vi "SPD.Liser Driver Test.vi"(8 "Error In":errorcluster, 11 "SPD.Stand Ctrl in":T1 {"spdDeviceSession"."hidSPD.Controller"."HV_bias" format="%#_6p, V"; "spdDeviceSession"."hidSPD.Controller"."TSet" format="%#_6p, DegC"}) -> (0 "Error Out":errorcluster, 1 "ok":bool, 2 "report":string, 3 "SPD.Stand Ctrl out":T1 {"spdDeviceSession"."hidSPD.Controller"."HV_bias" format="%#_6p, V"; "spdDeviceSession"."hidSPD.Controller"."TSet" format="%#_6p, DegC"})   [LabVIEW 2018]
uses:
  typedefs/SPD.Stand Ctrl.ctl
  Instruments/SPD HID Interface/hidSPDLibForLabView/LibVIs/hidSPD Controls/hidSPD Device Session.ctl
  Instruments/SPD HID Interface/hidSPDLibForLabView/LibVIs/hidSPD Controls/hidSPD Controller.ctl
  Instruments/KC705 DevBoard/typedefs/DevB.Session.ctl
  Instruments/KeySight 53230A/typedefs/FreqC.Session.ctl
  Instruments/KeySight 8164B/KeySight 8164B LAN InstrLib/typedefs/KeySight 8164B control.ctl
  Instruments/LeCroy SDA830/typedefs/LeCroy.Session.ctl
  typedefs/SPD.Events.ctl
  <vilib>/Utility/config.llb/Config Data RefNum.ctl
  typedefs/SPD.Meas Result.ctl
  Instruments/KeySight 8164B/KeySight 8164B LAN InstrLib/typedefs/KeySight 8164B Power Unit.ctl
  Instruments/KeySight 8164B/KeySight 8164B LAN InstrLib.lvlib
  Instruments/SPD HID Interface/hidSPDLibForLabView/hidSPDLibForLabView.lvlib
  <vilib>/Utility/config.llb/NI_LVConfig.lvlib
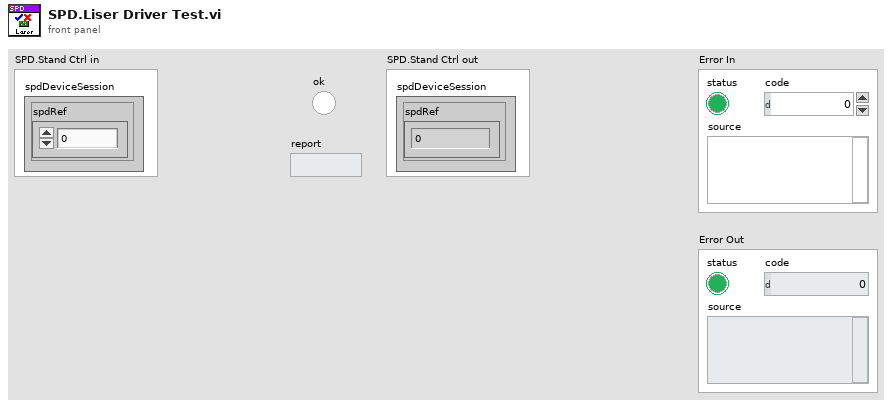
[diagram p1: front panel]
types:
  T1 = typedef "SPD.Stand Ctrl.ctl" = cluster{"spdDeviceSession":T2, "DevBSession":T4, "FreqCSession":T5, "8164BSession":T6, "LeCroySession":T7, "Events":T8, "configFile":T9, "SPD.Result":T10}
  T2 = typedef "hidSPDLibForLabView.lvlib/hidSPD Device Session.ctl" = cluster{"spdRef":u64, "connected":bool, "spdName":string, "hidSPD.Controller":T3}
  T3 = typedef "hidSPDLibForLabView.lvlib/hidSPD Controller.ctl" = cluster{"TSet":sgl, "HV_bias":sgl, "DDS_stb_code":u16}
  T4 = typedef "DevB.Session.ctl" = cluster{"DevBRef":refnum<visa-resource-name>, "connected":bool}
  T5 = typedef "FreqC.Session.ctl" = cluster{"FreqCRef":refnum<visa-resource-name>, "timeout":dbl, "Gate":dbl, "connected":bool}
  T6 = typedef "KeySight 8164B LAN InstrLib.lvlib/KeySight 8164B control.ctl" = cluster{"Connection ID":refnum<k5>, "Connected":bool, "Info":string, "Slots Info":string[]}
  T7 = typedef "LeCroy.Session.ctl" = cluster{"LeCroySession":refnum<visa-resource-name>, "connected":bool}
  T8 = typedef "SPD.Events.ctl" = cluster{"DCRTest":refnum<user-event>, "Stop":refnum<user-event>}
  T9 = typedef "NI_LVConfig.lvlib/Config Data RefNum.ctl" = refnum<k1>
  T10 = typedef "SPD.Meas Result.ctl" = cluster{"HV_Bias":dbl[][][], "Stb_code":dbl[], "Temprature":dbl[], "Data":dbl[][][][]}
  T11 = typedef "KeySight 8164B LAN InstrLib.lvlib/KeySight 8164B Power Unit.ctl" = enum16{"dBm", "Watt"}
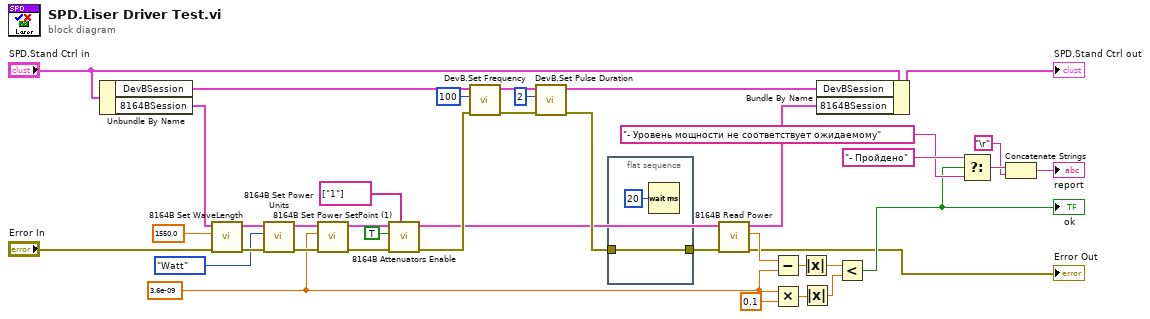
[diagram p0: block diagram]
diagram:
  w13 = 3.6e-09 ("Power Set Point")
  n1 = Unbundle By Name("SPD.Stand Ctrl in") -> ("DevBSession"=w30:T4, "8164BSession"=w26:T6)
  n2 = call "8164B Set WaveLength.vi"("error in"="Error In", "WaveLength, nm"=1550.0, "KeySight 8164B control in"=w26) -> ("error out"=w23:errorcluster, "KeySight 8164B control out"=w24:T6)  [unwired: 7 in]
  n3 = call "8164B Set Power Units.vi"("error in"=w23, "Power Unit"=KeySight_8164B_Power_Unit."Watt", "KeySight 8164B control in"=w24) -> ("error out"=w20:errorcluster, "KeySight 8164B control out"=w21:T6)  [unwired: 7 in]
  n4 = call "8164B Set Power SetPoint (1).vi"("error in"=w20, "Power Set Point"=w13, "KeySight 8164B control in"=w21) -> ("error out"=w5:errorcluster, "KeySight 8164B control out"=w6:T6)  [unwired: 7 in]
  n5 = call "8164B Attenuators Enable.vi"("Slots"=string[] ["1"], "error in"=w5, "Enable"=TRUE, "KeySight 8164B control in"=w6) -> ("error out"=w3:errorcluster, "KeySight 8164B control out"=w2:T6)  [unwired: 6 in]
  n6 = call "DevB.Set Frequency.vi"("error in (no error)"=w3, "Frequency"=100, "DevB Session in"=w30) -> ("error out"=w29:errorcluster, "DevB Session out"=w32:T4)  [unwired: 7 in]
  n7 = call "DevB.Set Pulse Duration.vi"("error in (no error)"=w29, "Pulse Duration"=2, "DevB Session in"=w32) -> ("error out"=w18:errorcluster, "DevB Session out"=w27:T4)  [unwired: 7 in]
  n8 = flat-sequence {
    tunnel: [w41] -> w17
    tunnel: w18 -> [w41]
    frame #0 {
      n9 = Wait (ms)(milliseconds to wait=u32 20) -> ()  [unwired: 1 out]
    }
  }
  n10 = call "8164B Read Power.vi"("error in"=w17, "KeySight 8164B control in"=w2) -> ("error out"=→"Error Out":errorcluster, "Power"=w15:dbl, "KeySight 8164B control out"=w16:T6)  [unwired: 7 in]
  n11 = Subtract(x=w15, y=w13) -> (x-y=w14:dbl)
  n12 = Multiply(x=w13, y=0.1) -> (x*y=w11:dbl)
  n13 = Absolute Value(x=w14) -> (abs(x)=w10:dbl)
  n14 = Absolute Value(x=w11) -> (abs(x)=w9:dbl)
  n15 = Bundle By Name(cluster="SPD.Stand Ctrl in", "DevBSession"=w27, "8164BSession"=w16) -> (→"SPD.Stand Ctrl out":T1)
  n16 = Less?(x=w10, y=w9) -> (x < y?=w8:bool)
  "ok" <- w8
  n17 = Select(t="- Пройдено" ("report"), s=w8, f="- Уровень мощности не соответствует ожидаемому") -> (s? t:f=w36:string)
  n18 = Concatenate Strings(w36, "\r") -> (→"report":string)
